vi "RF_Attn_send_command.vi"(1 "Value":dbl=3.0, 2 "Parameter":enum16{"Attenuation (dB)"}(ring), 3 "Insertion Loss":dbl=3.0, 4 "USB address":string="0:19") -> ()   [LabVIEW 2013]
uses:
  Attenuator_Vaunix-LDA_LabView_32Bit_Driver/Vaunix LDA/Vaunix LDA.lvlib
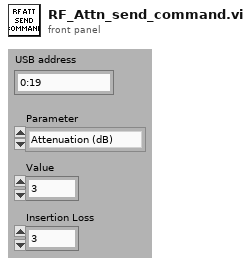
[diagram p1: front panel]
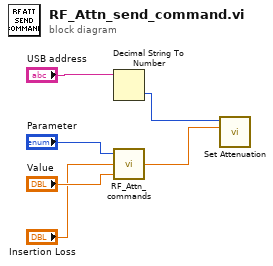
[diagram p0: block diagram]
diagram:
  n1 = Decimal String To Number(string="USB address") -> (number=w1:i32)  [unwired: 2 in, 1 out]
  n2 = call "RF_Attn_commands.vi"("Value"="Value", "Insertion Loss"="Insertion Loss", "Parameter"="Parameter") -> ("Command (dB)"=w3:dbl)
  n3 = call "Set Attenuation.vi"("Attenuation (dB)"=w3, "Device ID in"=w1) -> ()  [unwired: 8 in, 2 out]
